vi "Pack for gRPC.vi"(8 "error in":errorcluster, 9 "configuration / results":enum16{"Configuration", "Results"}(ring), 10 "data value":variant, 11 "measurement customizations in":refnum<class "Measurement Plugin.lvclass">) -> (0 "error out":errorcluster, 2 "any":T1, 3 "measurement customizations out":refnum<class "Measurement Plugin.lvclass">)   [LabVIEW 2022 SP3, in "Frequency Response.lvlib" / "Measurement Plugin.lvclass"]
uses:
  Measurement Plugin.lvclass
  <vilib>/gRPC/LabVIEW gRPC Library/Shared/Any.ctl
  C:/Program Files/National Instruments/LabVIEW 2022/vi.lib/Plug-In SDKs/Measurements/Measurement Plugin Service/Measurement Plugin Service.lvclass
  Measurement Configuration.ctl
  shared/controls/sweep profile.ctl
  Measurement Results.ctl
  2eca732d-dbaa-43bf-a7dd-ede2da65bc1b.vi
  a6012965-5700-4384-8228-972e71b6560c.vi
  <vilib>/gRPC/LabVIEW gRPC Library/Server API/Translate Protobuf Error.vi
  <vilib>/AdvancedString/1D String Array to Delimited String.vi
  <vilib>/gRPC/LabVIEW gRPC Library/Server API/Server/Get Server DLL Path.vi
  Frequency Response.lvlib
  <vilib>/Plug-In SDKs/Measurements/Measurement Plugin Service/Measurement Plugin Service.lvclass
  <vilib>/gRPC/LabVIEW gRPC Library/grpc-lvsupport-release.lvlib
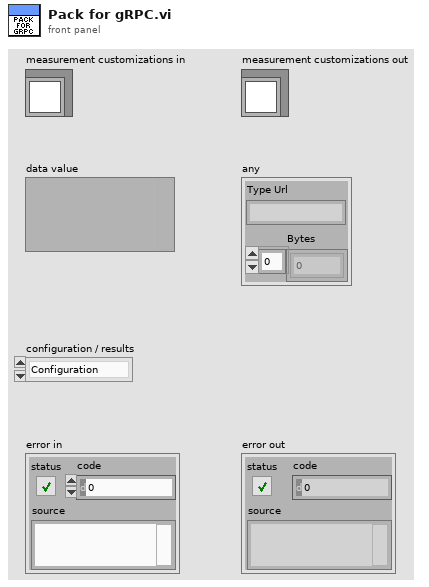
[diagram p1: front panel]
types:
  T1 = typedef "grpc-lvsupport-release.lvlib/Any.ctl" = cluster{"Type Url":string, "Bytes":u8[]}
  T2 = typedef "grpc-lvsupport-release.lvlib/grpcId.ctl" = u64
  T3 = typedef "Frequency Response.lvlib/Measurement Configuration.ctl" = cluster{"digital channel list":string, "input cfg file":string, "digital mic sensitivity (dBFS)":dbl, "ref mic channel":string, "ref mic sensitivity (mV/Pa)":dbl, "output channel":string, "output level (dBSPL)":dbl, "output voltage ratio":dbl, "start frequency":dbl, "stop frequency":dbl, "number of steps":dbl, "sweep profile":T4}
  T4 = typedef "sweep profile.ctl" = enum32{"Linear", "Logarithmic"}
  T5 = typedef "Frequency Response.lvlib/Measurement Results.ctl" = cluster{"channel name":string, "frequency (Hz)":dbl[], "amplitude (dBr)":dbl[], "THD+N":dbl[], "THD":dbl[], "wfm - dt":dbl, "wfm - data":dbl[], "ref mic wfm - dt":dbl, "ref mic wfm - data":dbl[]}
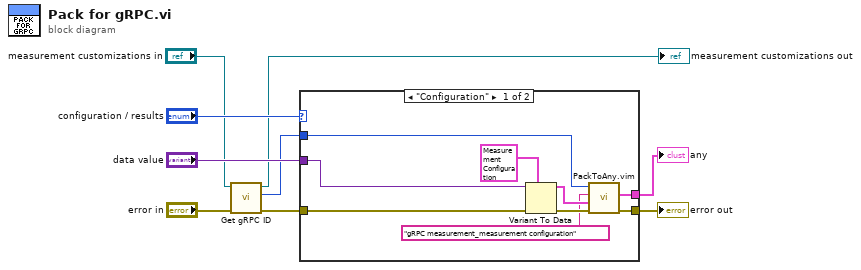
[diagram p0: block diagram]
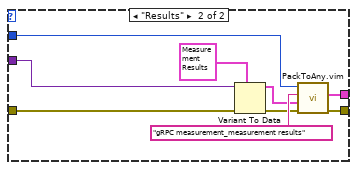
[diagram p2: hidden frame]
diagram:
  n1 = call <vilib>:"Get gRPC ID.vi"("error in"="error in", "measurement plugin service in"="measurement customizations in") -> ("error out"=w4:errorcluster, "gRPC ID"=w1:T2, "measurement plugin service out"=→"measurement customizations out":refnum<class "Measurement Plugin.lvclass">)  [unwired: 7 in]
  n2 = case shown="\"Configuration\"" "configuration / results" {
    tunnel: w4 -> [w18 w27]
    tunnel: "data value" -> [w17 w26]
    tunnel: w1 -> [w14 w22]
    tunnel: [w16 w24] -> w8
    tunnel: [w15 w23] -> w7
    frame "Configuration" {
      n3 = Variant To Data(error in=w18, type=T3 {"digital channel list"="Lorem ipsum dolor sit", "input cfg file"="", "digital mic sensitivity (dBFS)"=1.2, "ref mic channel"="PXI1Slot3/ai0", "ref mic sensitivity (mV/Pa)"=32.0, "output channel"="PXI1Slot3/ao0", "output level (dBSPL)"=64.0, "output voltage ratio"=-32.0, "start frequency"=-64.0, "stop frequency"=-64.0, "number of steps"=1.0, "sweep profile"=enum."Logarithmic"} ("measurement configuration"), Variant=w17) -> (data=w13:T3, error out=w12:errorcluster)
      n4 = call "PackToAny.vim"("error in"=w12, "Data To Pack"=w13, "Message Type"="gRPC measurement_measurement configuration", "gRPCid in"=w14) -> ("error out"=w16:errorcluster, "Any"=w15:T1)  [unwired: 5 in, 1 out]
    }
    frame "Results" {
      n5 = Variant To Data(error in=w27, type=T5 {"channel name"="Empty", "frequency (Hz)"=[], "amplitude (dBr)"=[], "THD+N"=[], "THD"=[0.0], "wfm - dt"=0.0, "wfm - data"=[0.0], "ref mic wfm - dt"=0.0, "ref mic wfm - data"=[0.0]} ("Measurement Results"), Variant=w26) -> (data=w20:T5, error out=w19:errorcluster)
      n6 = call "PackToAny.vim"("error in"=w19, "Data To Pack"=w20, "Message Type"="gRPC measurement_measurement results", "gRPCid in"=w22) -> ("error out"=w24:errorcluster, "Any"=w23:T1)  [unwired: 5 in, 1 out]
    }
  }
  "error out" <- w8
  "any" <- w7
